vi "ROI entry-Previous ROI compat-Zoom.vi"(8 "error in (no error)":errorcluster, 9 "Proceed":bool=TRUE, 11 "Old ROI file path":path) -> (0 "error out":errorcluster, 1 "Proceed":bool, 3 "Old ROI file path (dup)":path)   [LabVIEW 2020]
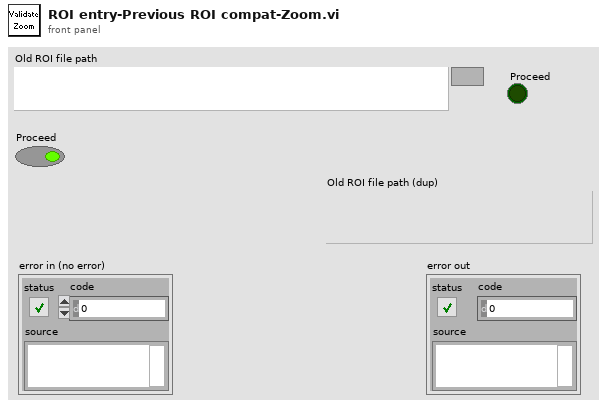
[diagram p1: front panel]
types:
  T1 = typedef "Fixed strings.ctl" = cluster{"ROI file name":string, "Normalised ROI file name":string, "Zplane Pockels values file name":string, "Functional data folder name":string, "Experiment Header file name":string, "Z-stack images folder name":string, "Groups setup rel. path":string, "Groups text file rel. path":string, "TDMS files folder name (F.img)":string, "TDMS files folder name (V.acq)":string, "TDMS files folder name (Pl.acq)":string, "Cycle rel times sequence file":string, "Dynamically called VIs folder name":string, "Time Series folder base name":string, "Parameter Sweep":string, "Calibration Profile Images":string}
  T2 = typedef "AOL_Globals.ctl" = cluster{"Imaging Protocol":T3, "Number of POI":u16, "Number of Miniscans":u16, "Number of Trials":u16, "Number of Cycles ":u64, "# Averaged Frames":u16, "Laser power (%)":u8, "Pockels (V)":dbl, "Acquisition Length (sec)":dbl, "Fill time (us)":dbl, "POI Dwell time (us)":dbl, "Miniscan Dwell time per pixel (us)":dbl, "PMT 1":dbl, "PMT 2":dbl, "Back Apperture (mA)":dbl, "Frame Size":T4, "Center Frequency":dbl, "Field of View (um)":dbl, "Field of View (norm)":dbl, "DwellTime (us)":dbl, "Ref Dwell Time (us)":dbl, "Wavelength (nm)":dbl, "Zoom":dbl, "AOL Z":dbl, "AOL Mode":T5, "GridXY":dbl, "GridZ":dbl, "TriggerPeriod (sec)":dbl, "Number of Pixels in Miniscan":u16, "Experiment folder path":path, "X centre":dbl, "Y centre":dbl, "Angle (degrees)":dbl, "Angle Xs (degrees)":dbl, "Angle Ys (degrees)":dbl, "Plane Mode":T6, "Threshold":u16[], "Regenerate Chirps":bool, "Rectangle ROI length (pixels)":u16, "Rectangle ROI height (pixels)":u16, "AOD fill":u16, "StartupDelay":i32, "Samples Wait after Trigger":u16, "Slip Cycle":u32, "Add Cycle":bool, "Functional Mode":T7, "Z Start":dbl, "Z Stop":dbl, "# Planes":i32, "Total Pixels":i32, "Variable Miniscan Pixels":u16[], "Use Variable Length":bool, "Use Variable Resolution":bool, "Laser power (%) at Z Start":u8, "Laser power (%) at Z Stop":u8, "Ref Z Step":i8}
  T3 = typedef "Imaging Protocols enum.ctl" = enum16{"AOL Z-Stack", "Motor Z Stack", "Parameter Sweep", "Functional Acquisition", "Single Plane Acquisition", "Volume Acquisition", "Live Imaging", "Live Plane Imaging", "Live Volume Imaging"}
  T4 = typedef "Frame Size.ctl" = u16
  T5 = typedef "AOL modes.ctl" = enum16{"Raster", "Structural", "Pointing", "Mini Scan", "Alignment"}
  T6 = typedef "Plane Mode.ctl" = u16
  T7 = typedef "Functional Mode.ctl" = enum16{"Point", "Line", "Patch", "Plane", "Volume"}
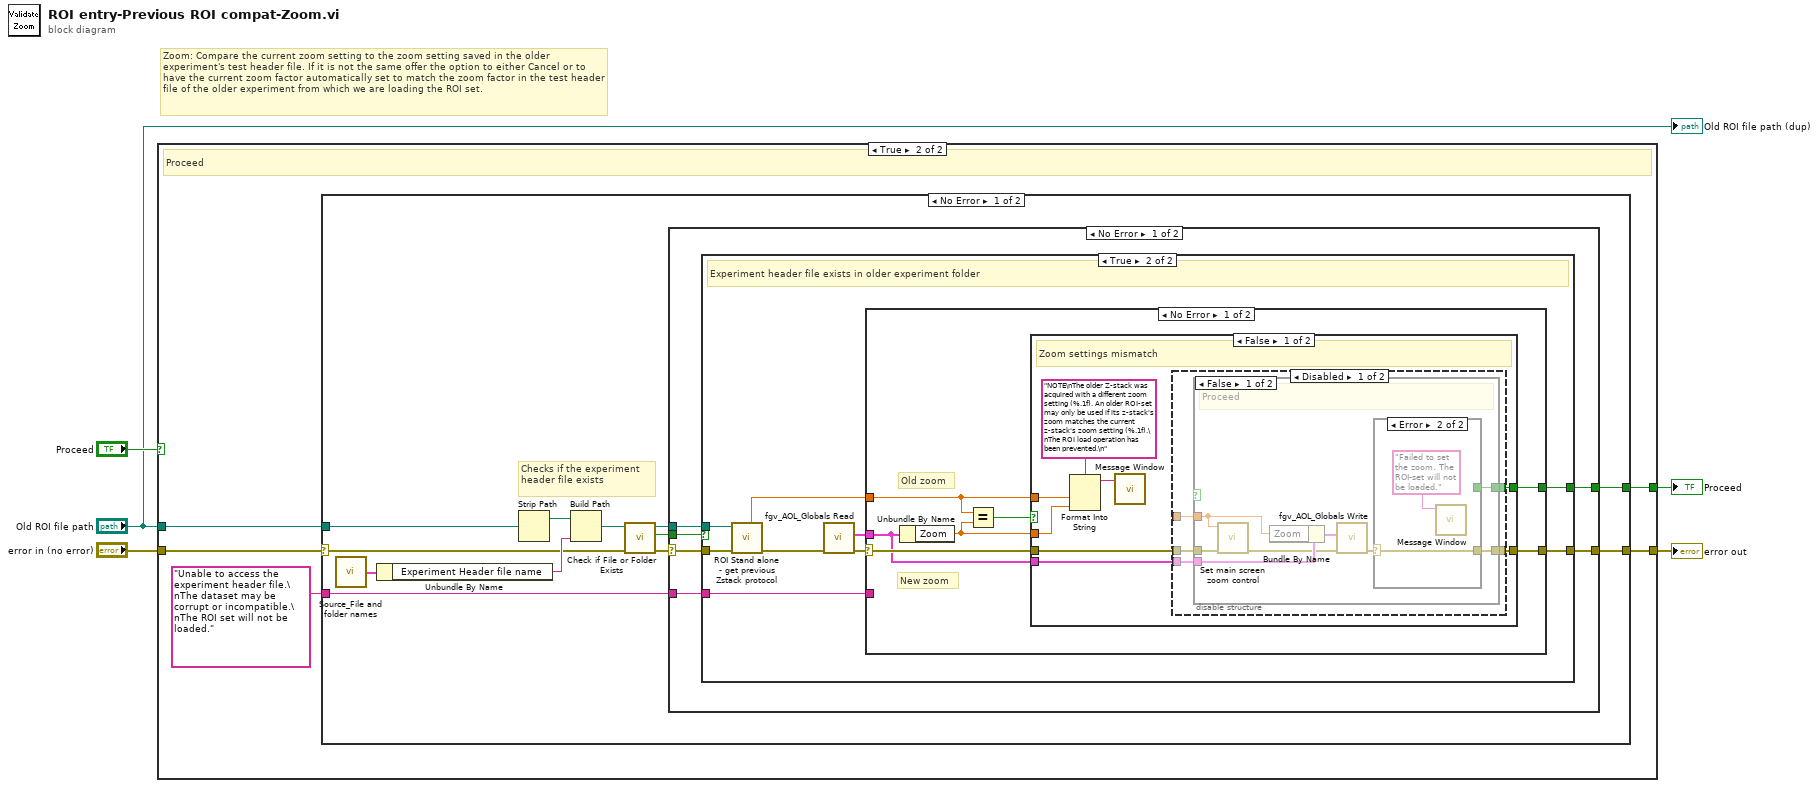
[diagram p0: block diagram]
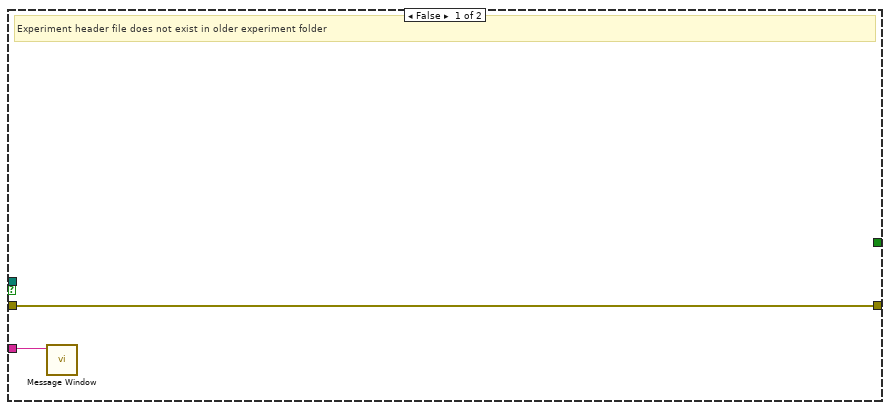
[diagram p3: hidden frame]
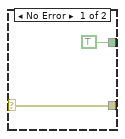
[diagram p4: hidden frame]
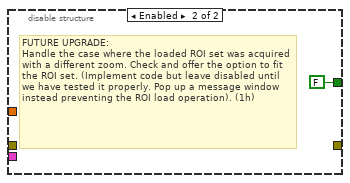
[diagram p6: hidden frame]
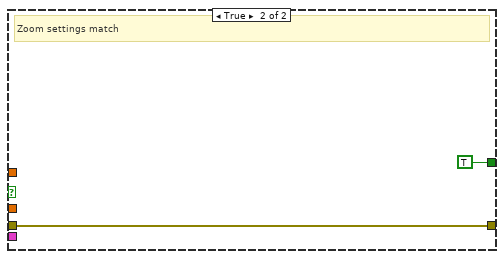
[diagram p7: hidden frame]
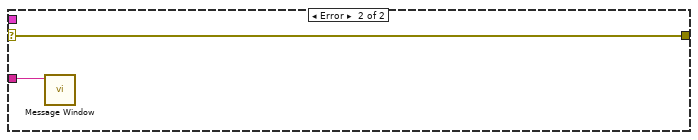
[diagram p8: hidden frame]
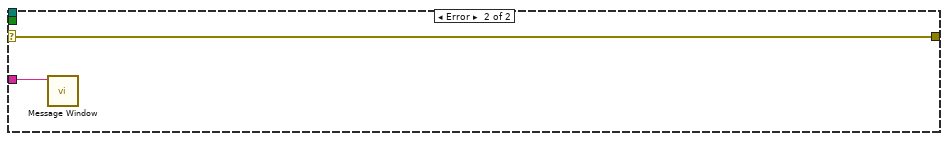
[diagram p9: hidden frame]
diagram:
  # "Zoom: Compare the current zoom setting to the zoom setting saved in the older experiment's test header file. If it is not the same offer the option to either Cancel or to have the current zoom factor automatically set to match the zoom factor in the test header file of the older experiment from which we are loading the ROI set."
  n1 = case shown="True" "Proceed" {
    tunnel: "Old ROI file path" -> [_ w11]
    tunnel: [w6 w9] -> w5
    tunnel: "error in (no error)" -> [w6 w8]
    tunnel: [_ w7] -> w3
    frame False {
      # "Skip"
    }
    frame True {
      # "Proceed"
      n2 = case shown="No Error" w8 {
        selector: w8 -> [w14 w81]
        tunnel: w11 -> [w21 _]
        tunnel: [w17 _] -> w7
        tunnel: [w13 w81] -> w9
        tunnel: "Unable to access the experiment header file.\nThe dataset may be corrupt or incompatible.\nThe ROI set will not be loaded." ("Message string") -> [w12 _]
        frame No Error {
          # "Checks if the experiment header file exists"
          n3 = call "Source_File and folder names.vi"() -> ("Fixed strings"=w22:T1)  [unwired: 1 in]
          n4 = Unbundle By Name(w22) -> ("Experiment Header file name"=w19:string)
          n5 = Strip Path(path=w21) -> (stripped path=w20:path)  [unwired: 1 out]
          n6 = Build Path(base path=w20, name or relative path=w19) -> (appended path=w23:path)
          n7 = call <vilib>:"Check if File or Folder Exists.vi"("error in (no error)"=w14, "path"=w23) -> ("error out"=w15:errorcluster, "file or folder exists?"=w18:bool, "dup path"=w16:path)  [unwired: 7 in]
          n8 = case shown="No Error" w15 {
            selector: w15 -> [w26 w80]
            tunnel: w18 -> [w29 _]
            tunnel: [w28 _] -> w17
            tunnel: w16 -> [w27 _]
            tunnel: [w25 w80] -> w13
            tunnel: w12 -> [w24 w79]
            frame No Error {
              n9 = case shown="True" w29 {
                tunnel: [_ w39] -> w28
                tunnel: w27 -> [_ w34]
                tunnel: w26 -> [w31 w35]
                tunnel: [w31 w38] -> w25
                tunnel: w24 -> [w30 w36]
                frame False {
                  # "Experiment header file does not exist in older experiment folder"
                  n10 = call "Message Window.vi"("Message string"=w30) -> ()  [unwired: 10 in, 1 out]
                }
                frame True {
                  # "Experiment header file exists in older experiment folder"
                  n11 = call "ROI Stand alone - get previous Zstack protocol.vi"("error in (no error)"=w35, "path"=w34) -> ("error out"=w33:errorcluster, "zoom"=w32:dbl)  [unwired: 5 in, 3 out]
                  n12 = call "fgv_AOL_Globals Read.vi"("error in (no error)"=w33) -> ("error out"=w37:errorcluster, "AOL_Globals"=w40:T2)  [unwired: 8 in, 1 out]
                  n13 = case shown="No Error" w37 {
                    selector: w37 -> [w45 w78]
                    tunnel: w40 -> [w44 _]
                    tunnel: [w47 _] -> w39
                    tunnel: [w46 w78] -> w38
                    tunnel: w36 -> [_ w77]
                    tunnel: w32 -> [w41 _]
                    frame No Error {
                      # "New zoom"
                      # "Old zoom"
                      n14 = Unbundle By Name(w44) -> ("Zoom"=w43:dbl)
                      n15 = Equal?(x=w41, y=w43) -> (x = y?=w42:bool)
                      n16 = case shown="False" w42 {
                        tunnel: [w55 TRUE] -> w47
                        tunnel: w45 -> [w54 w75]
                        tunnel: [w53 w75] -> w46
                        tunnel: w44 -> [w52 _]
                        tunnel: w43 -> [w50 _]
                        tunnel: w41 -> [w48 _]
                        frame False {
                          # "Zoom settings mismatch"
                          n17 = Format Into String(format string="NOTE\nThe older Z-stack was acquired with a different zoom setting (%.1f). An older ROI-set may only be used if its z-stack's zoom matches the current z-stack's zoom setting (%.1f).\nThe ROI load operation has been prevented.\n" ("Message string"), w48, w50) -> (resulting string=w49:string)  [unwired: 2 in, 1 out]
                          n18 = call "Message Window.vi"("Message string"=w49) -> ()  [unwired: 10 in, 1 out]
                          n19 = disable-structure shown="Disabled" {
                            disable-tunnel: [w60 FALSE] -> w55
                            disable-tunnel: _ -> [w59 _]
                            disable-tunnel: w54 -> [w58 _]
                            disable-tunnel: [w57 _] -> w53
                            disable-tunnel: w52 -> [w56 _]
                            frame Disabled {
                              n20 = case shown="False" {
                                selector: _ -> [_ _]
                                tunnel: [w68 _] -> w60
                                tunnel: w59 -> [w65 _]
                                tunnel: w58 -> [w64 w73]
                                tunnel: [w61 w73] -> w57
                                tunnel: w56 -> [w67 _]
                                frame False {
                                # "Proceed"
                                n21 = call "Set main screen zoom control.vi"("error in (no error)"=w64, "Zoom"=w65) -> ("error out"=w63:errorcluster)  [unwired: 9 in]
                                n22 = Bundle By Name(cluster=w67, "Zoom"=w65) -> (w66:T2)
                                n23 = call "fgv_AOL_Globals Write.vi"("error in (no error)"=w63, "AOL_Globals"=w66) -> ("error out"=w62:errorcluster)  [unwired: 9 in]
                                n24 = case shown="Error" w62 {
                                selector: w62 -> [w69 w72]
                                tunnel: [TRUE _] -> w68
                                tunnel: [w69 w72] -> w61
                                frame No Error {
                                }
                                frame Error {
                                n25 = call "Message Window.vi"("Message string"="Failed to set the zoom. The ROI-set will not be loaded.") -> ()  [unwired: 10 in, 1 out]
                                }
                                }
                                }
                                frame True {
                                # "Cancelled"
                                }
                              }
                            }
                            frame Enabled {
                              # "FUTURE UPGRADE:\nHandle the case where the loaded ROI set was acquired with a different zoom. Check and offer the option to fit the ROI set. (Implement code but leave disabled until we have tested it properly. Pop up a message window instead preventing the ROI load operation). (1h)"
                            }
                          }
                        }
                        frame True {
                          # "Zoom settings match"
                        }
                      }
                    }
                    frame Error {
                      n26 = call "Message Window.vi"("Message string"=w77) -> ()  [unwired: 10 in, 1 out]
                    }
                  }
                }
              }
            }
            frame Error {
              n27 = call "Message Window.vi"("Message string"=w79) -> ()  [unwired: 10 in, 1 out]
            }
          }
        }
        frame Error {
        }
      }
    }
  }
  "error out" <- w5
  "Proceed" <- w3
  "Old ROI file path (dup)" <- "Old ROI file path"
